vi "Lift Logic.vi"(0 "Manual Up":bool, 1 "Manual Down":bool, 2 "Climb Actuation":bool, 3 "Load":bool, 4 "Switch":bool, 5 "Exchange":bool, 6 "Scale Low":bool, 7 "Scale Mid":bool, 8 "Reset State Machine":bool, 9 "Scale High":bool, 11 "Stow":bool, 13 "Climb":bool, 15 "Visited Disabled":bool) -> (12 "Open Arms":bool, 14 "Reset Arm":bool, 16 "Portal Out":bool, 17 "Climb Out":bool, 18 "Manual Up Out":bool, 19 "Stow Out":bool, 20 "Manual Down Out":bool, 21 "Climb Actuation Out":bool, 22 "Load Out":bool, 23 "Switch Out":bool, 24 "Exchange Out":bool, 25 "Scale Low Out":bool, 26 "Scale Mid Out":bool, 27 "Scale High Out":bool)   [LabVIEW 2017]
uses:
  Lift Portal Switch Setpoints.ctl
panel:
  in  "Portal":bool
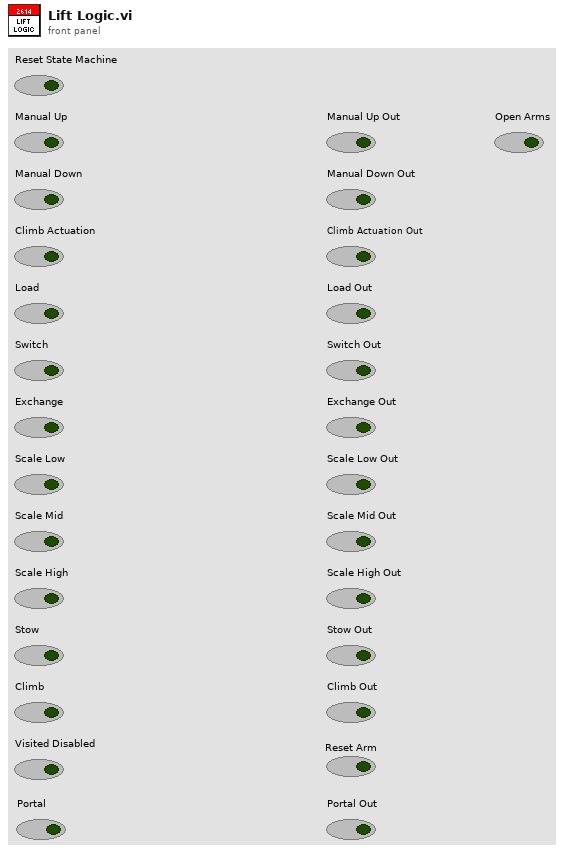
[diagram p1: front panel]
types:
  T1 = typedef "Lift Portal Switch Setpoints.ctl" = enum16{"Waiting for First", "Load", "Portal"}
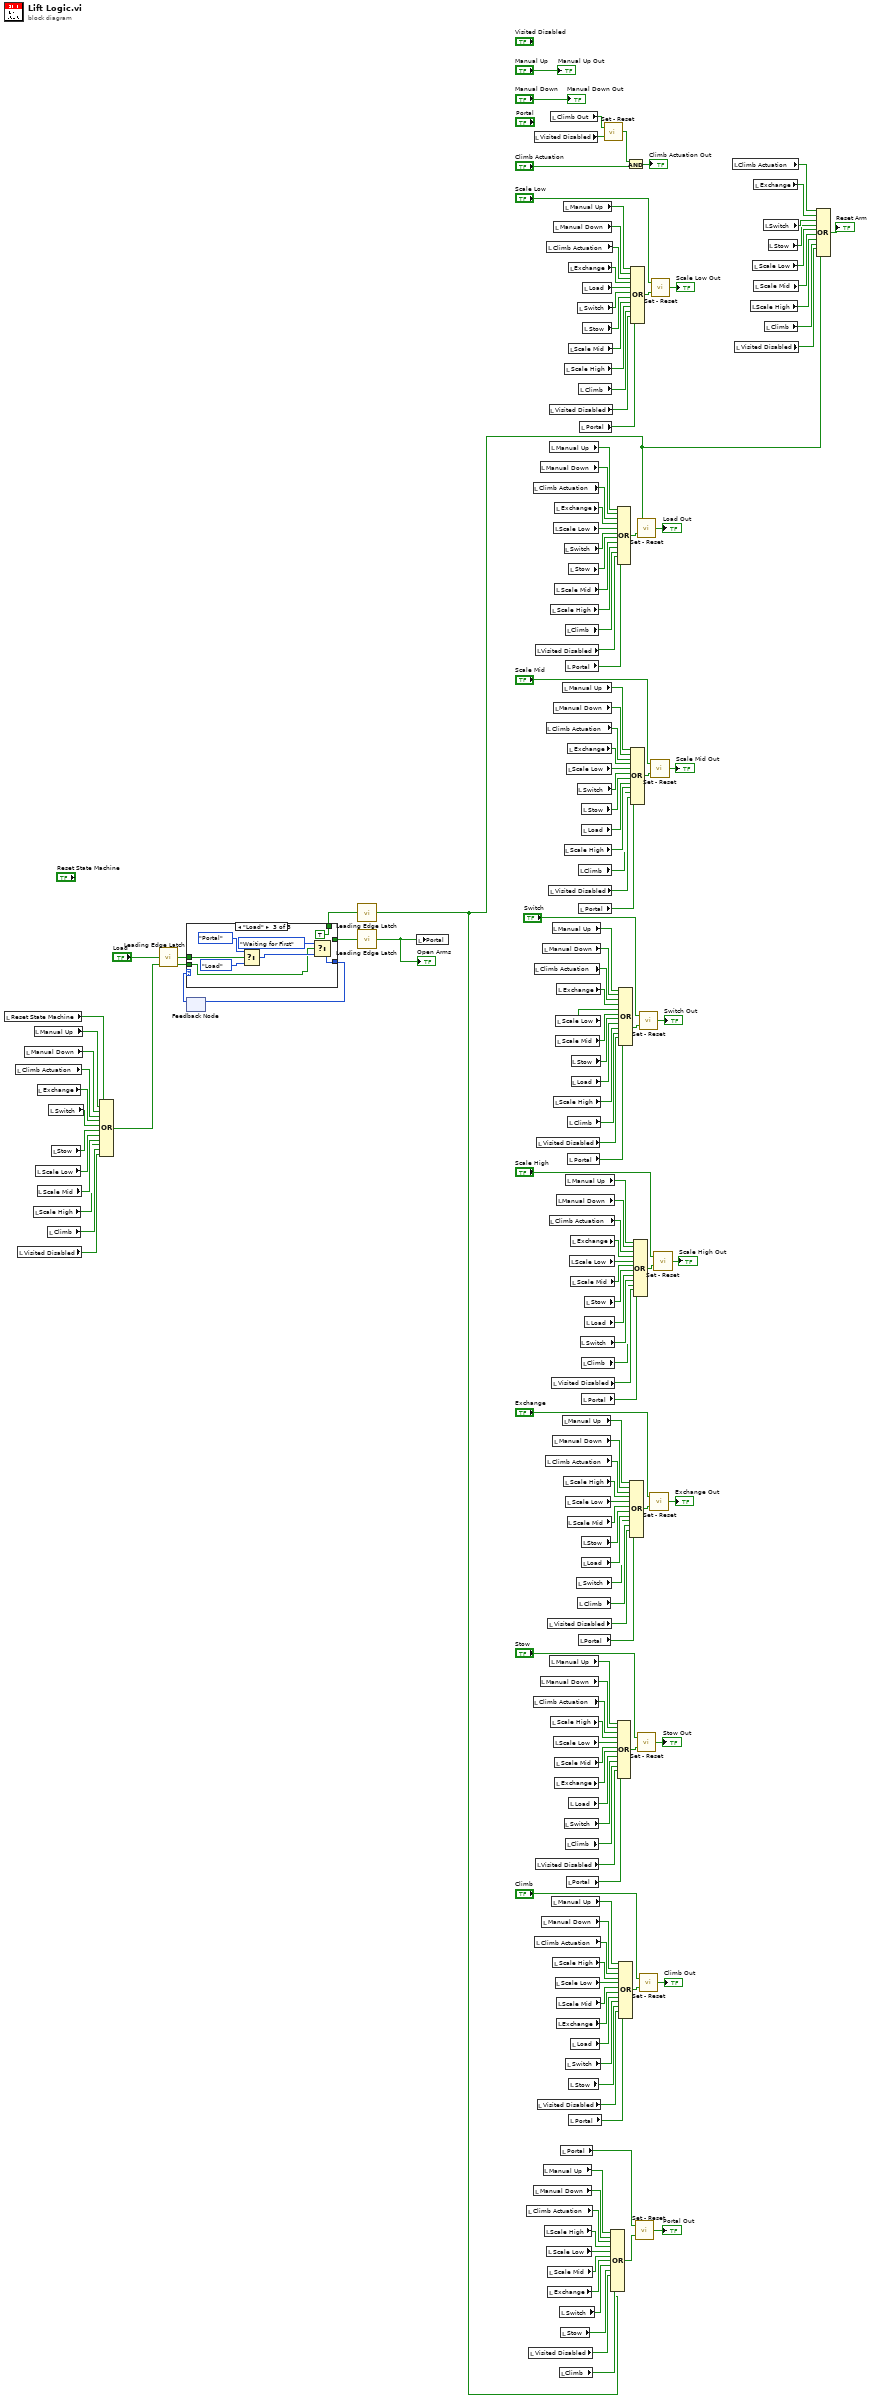
[diagram p0: block diagram]
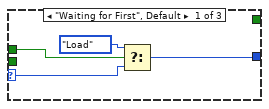
[diagram p2: hidden frame]
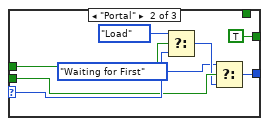
[diagram p3: hidden frame]
diagram:
  n1 = local read "Reset State Machine"() -> (w2:bool)
  n2 = local read "Climb Actuation"() -> (w22:bool)
  n3 = local read "Visited Disabled"() -> (w17:bool)
  n4 = local read "Manual Down"() -> (w4:bool)
  n5 = local read "Scale High"() -> (w19:bool)
  n6 = local read "Manual Up"() -> (w3:bool)
  n7 = local read "Scale Low"() -> (w21:bool)
  n8 = local read "Exchange"() -> (w23:bool)
  n9 = local read "Scale Mid"() -> (w20:bool)
  n10 = local read "Climb"() -> (w18:bool)
  n11 = local read "Switch"() -> (w24:bool)
  n12 = local read "Stow"() -> (w25:bool)
  n13 = Compound Arithmetic op=OR(w2, w3, w4, w22, w23, w24, w25, w21, w20, w19, w18, w17) -> (w15:bool)
  n14 = call "Leading Edge Latch.vi"("Input"="Load") -> ("Output"=w16:bool)
  n15 = feedback #1() -> (w9:T1)  [unwired: 1 in]
  n16 = case shown="\"Load\"" w9 {
    selector: w9 -> [w173 w182 _]
    tunnel: w16 -> [w174 w183 w188]
    tunnel: w15 -> [_ w181 w184]
    tunnel: [_ TRUE _] -> w7
    tunnel: [_ _ TRUE] -> w13
    tunnel: [w172 w177 w185] -> w10
    frame "Waiting for First", Default {
      n17 = Select(t=Lift_Portal_Switch_Setpoints."Load" ("Portal-Switch"), s=w174, f=w173) -> (s? t:f=w172:T1)
    }
    frame "Portal" {
      n18 = Select(t=Lift_Portal_Switch_Setpoints."Load", s=w183, f=w182) -> (s? t:f=w180:T1)
      n19 = Select(t=Lift_Portal_Switch_Setpoints."Waiting for First", s=w181, f=w180) -> (s? t:f=w177:T1)
    }
    frame "Load" {
      n20 = Select(t=Lift_Portal_Switch_Setpoints."Portal" ("Portal-Switch"), s=w188, f=Lift_Portal_Switch_Setpoints."Load") -> (s? t:f=w186:T1)
      n21 = Select(t=Lift_Portal_Switch_Setpoints."Waiting for First", s=w184, f=w186) -> (s? t:f=w185:T1)
    }
  }
  n22 = feedback-in #1(w10) -> ()
  n23 = call "Leading Edge Latch.vi"("Input"=w13) -> ("Output"=w6:bool)
  n24 = call "Leading Edge Latch.vi"("Input"=w7) -> ("Output"=w1:bool)
  "Open Arms" <- w1
  n25 = local write "Portal"(w1) -> ()
  n26 = local read "Climb Actuation"() -> (w38:bool)
  n27 = local read "Visited Disabled"() -> (w35:bool)
  n28 = local read "Climb Actuation"() -> (w111:bool)
  n29 = local read "Climb Actuation"() -> (w125:bool)
  n30 = local read "Manual Down"() -> (w37:bool)
  n31 = local read "Visited Disabled"() -> (w58:bool)
  n32 = local read "Climb Actuation"() -> (w134:bool)
  n33 = local read "Climb Actuation"() -> (w122:bool)
  n34 = local read "Visited Disabled"() -> (w146:bool)
  n35 = local read "Visited Disabled"() -> (w154:bool)
  n36 = local read "Visited Disabled"() -> (w148:bool)
  n37 = local read "Visited Disabled"() -> (w157:bool)
  n38 = local read "Manual Down"() -> (w137:bool)
  n39 = local read "Manual Down"() -> (w126:bool)
  n40 = local read "Manual Down"() -> (w123:bool)
  n41 = local read "Manual Down"() -> (w135:bool)
  n42 = local read "Manual Up"() -> (w36:bool)
  n43 = local read "Scale High"() -> (w44:bool)
  n44 = local read "Climb Actuation"() -> (w128:bool)
  n45 = local read "Climb Actuation"() -> (w139:bool)
  n46 = local read "Climb Actuation"() -> (w142:bool)
  n47 = local read "Scale Low"() -> (w43:bool)
  n48 = local read "Visited Disabled"() -> (w152:bool)
  n49 = local read "Scale Mid"() -> (w42:bool)
  n50 = local read "Exchange"() -> (w41:bool)
  n51 = local read "Visited Disabled"() -> (w147:bool)
  n52 = local read "Visited Disabled"() -> (w145:bool)
  n53 = local read "Climb Actuation"() -> (w131:bool)
  n54 = local read "Manual Up"() -> (w138:bool)
  n55 = local read "Manual Up"() -> (w127:bool)
  n56 = local read "Climb Out"() -> (w59:bool)
  n57 = local read "Scale High"() -> (w105:bool)
  n58 = local read "Scale High"() -> (w73:bool)
  n59 = local read "Visited Disabled"() -> (w150:bool)
  n60 = local read "Manual Up"() -> (w124:bool)
  n61 = local read "Manual Up"() -> (w136:bool)
  n62 = local read "Manual Down"() -> (w129:bool)
  n63 = local read "Scale High"() -> (w60:bool)
  n64 = local read "Scale Low"() -> (w109:bool)
  n65 = local read "Manual Down"() -> (w140:bool)
  n66 = local read "Scale High"() -> (w90:bool)
  n67 = local read "Scale Low"() -> (w72:bool)
  n68 = local read "Manual Down"() -> (w143:bool)
  n69 = local read "Exchange"() -> (w110:bool)
  n70 = local read "Scale Mid"() -> (w106:bool)
  n71 = local read "Scale Mid"() -> (w71:bool)
  n72 = local read "Exchange"() -> (w70:bool)
  n73 = local read "Scale Low"() -> (w61:bool)
  n74 = local read "Scale Low"() -> (w94:bool)
  n75 = local read "Scale Mid"() -> (w93:bool)
  n76 = local read "Manual Down"() -> (w132:bool)
  n77 = local read "Scale Mid"() -> (w62:bool)
  n78 = local read "Exchange"() -> (w63:bool)
  n79 = local read "Exchange"() -> (w95:bool)
  n80 = local read "Climb"() -> (w12:bool)
  n81 = local read "Switch"() -> (w40:bool)
  n82 = local read "Portal"() -> (w14:bool)
  n83 = local read "Stow"() -> (w39:bool)
  n84 = local read "Manual Up"() -> (w130:bool)
  n85 = local read "Manual Up"() -> (w141:bool)
  n86 = local read "Manual Up"() -> (w144:bool)
  n87 = local read "Scale High"() -> (w80:bool)
  n88 = local read "Switch"() -> (w108:bool)
  n89 = local read "Scale High"() -> (w97:bool)
  n90 = local read "Switch"() -> (w68:bool)
  n91 = local read "Scale High"() -> (w113:bool)
  n92 = local read "Climb"() -> (w104:bool)
  n93 = local read "Climb"() -> (w67:bool)
  n94 = local read "Portal"() -> (w27:bool)
  n95 = local read "Manual Up"() -> (w133:bool)
  n96 = local read "Scale Low"() -> (w79:bool)
  n97 = local read "Switch"() -> (w65:bool)
  n98 = local read "Scale Low"() -> (w101:bool)
  n99 = local read "Portal"() -> (w32:bool)
  n100 = local read "Scale Mid"() -> (w78:bool)
  n101 = local read "Exchange"() -> (w102:bool)
  n102 = local read "Climb"() -> (w89:bool)
  n103 = local read "Portal"() -> (w29:bool)
  n104 = local read "Exchange"() -> (w118:bool)
  n105 = local read "Scale Mid"() -> (w114:bool)
  n106 = local read "Stow"() -> (w107:bool)
  n107 = local read "Load"() -> (w69:bool)
  n108 = local read "Stow"() -> (w66:bool)
  n109 = local read "Portal"() -> (w33:bool)
  n110 = local read "Scale Low"() -> (w86:bool)
  n111 = local read "Exchange"() -> (w87:bool)
  n112 = local read "Scale Mid"() -> (w85:bool)
  n113 = local read "Load"() -> (w64:bool)
  n114 = local read "Stow"() -> (w92:bool)
  n115 = local read "Load"() -> (w91:bool)
  n116 = local read "Switch"() -> (w75:bool)
  n117 = local read "Switch"() -> (w100:bool)
  n118 = local read "Switch"() -> (w116:bool)
  n119 = local read "Climb"() -> (w74:bool)
  n120 = local read "Climb"() -> (w96:bool)
  n121 = local read "Portal"() -> (w31:bool)
  n122 = local read "Climb"() -> (w112:bool)
  n123 = local read "Portal"() -> (w28:bool)
  n124 = local read "Portal"() -> (w26:bool)
  n125 = local read "Switch"() -> (w82:bool)
  n126 = local read "Climb"() -> (w81:bool)
  n127 = local read "Stow"() -> (w77:bool)
  n128 = local read "Load"() -> (w76:bool)
  n129 = local read "Stow"() -> (w99:bool)
  n130 = local read "Load"() -> (w98:bool)
  n131 = local read "Portal"() -> (w30:bool)
  n132 = local read "Load"() -> (w117:bool)
  n133 = local read "Stow"() -> (w115:bool)
  n134 = local read "Stow"() -> (w84:bool)
  n135 = local read "Load"() -> (w83:bool)
  n136 = call "Set - Reset.vi"("Reset"=w58, "Set"=w59) -> ("Output"=w57:bool)
  n137 = Compound Arithmetic op=OR(w36, w37, w38, w44, w43, w42, w41, w40, w39, w35, w12, w12, w6) -> (w34:bool)
  n138 = Compound Arithmetic op=OR(w138, w137, w111, w110, w109, w108, w107, w106, w105, w104, w146, w27) -> (w121:bool)
  n139 = Compound Arithmetic op=OR(w127, w126, w125, w73, w72, w71, w70, w69, w68, w67, w154, w32) -> (w156:bool)
  n140 = Compound Arithmetic op=OR(w136, w135, w134, w95, w94, w93, w92, w91, w90, w89, w148, w29) -> (w119:bool)
  n141 = Compound Arithmetic op=OR(w124, w123, w122, w60, w61, w62, w63, w64, w65, w66, w157, w33) -> (w163:bool)
  n142 = And(x=w57, y="Climb Actuation") -> (x .and. y?=→"Climb Actuation Out":bool)
  n143 = Compound Arithmetic op=OR(w130, w129, w128, w80, w79, w78, w77, w76, w75, w74, w152, w31) -> (w151:bool)
  n144 = Compound Arithmetic op=OR(w141, w140, w139, w102, w101, w100, w99, w98, w97, w96, w147, w28) -> (w120:bool)
  n145 = Compound Arithmetic op=OR(w144, w143, w142, w118, w117, w116, w115, w114, w113, w112, w145, w26) -> (w161:bool)
  n146 = Compound Arithmetic op=OR(w133, w132, w131, w87, w86, w85, w84, w83, w82, w81, w150, w30) -> (w149:bool)
  n147 = call "Set - Reset.vi"("Reset"=w34, "Set"=w14) -> ("Output"=→"Portal Out":bool)
  n148 = call "Set - Reset.vi"("Reset"=w121, "Set"=w6) -> ("Output"=→"Load Out":bool)
  n149 = call "Set - Reset.vi"("Reset"=w156, "Set"="Stow") -> ("Output"=→"Stow Out":bool)
  n150 = call "Set - Reset.vi"("Reset"=w119, "Set"="Switch") -> ("Output"=→"Switch Out":bool)
  n151 = call "Set - Reset.vi"("Reset"=w163, "Set"="Climb") -> ("Output"=→"Climb Out":bool)
  n152 = call "Set - Reset.vi"("Reset"=w151, "Set"="Exchange") -> ("Output"=→"Exchange Out":bool)
  n153 = call "Set - Reset.vi"("Reset"=w120, "Set"="Scale Mid") -> ("Output"=→"Scale Mid Out":bool)
  n154 = call "Set - Reset.vi"("Reset"=w161, "Set"="Scale Low") -> ("Output"=→"Scale Low Out":bool)
  n155 = call "Set - Reset.vi"("Reset"=w149, "Set"="Scale High") -> ("Output"=→"Scale High Out":bool)
  n156 = local read "Climb Actuation"() -> (w49:bool)
  n157 = local read "Visited Disabled"() -> (w54:bool)
  n158 = local read "Scale High"() -> (w52:bool)
  n159 = local read "Scale Low"() -> (w50:bool)
  n160 = local read "Exchange"() -> (w48:bool)
  n161 = local read "Scale Mid"() -> (w51:bool)
  n162 = local read "Switch"() -> (w47:bool)
  n163 = local read "Climb"() -> (w53:bool)
  n164 = local read "Stow"() -> (w46:bool)
  n165 = Compound Arithmetic op=OR(w49, w48, w47, w46, w50, w51, w52, w53, w54, w6) -> (→"Reset Arm":bool)
  "Manual Up Out" <- "Manual Up"
  "Manual Down Out" <- "Manual Down"
